vi "Aplicaderiva.vi"() -> ()   [LabVIEW 2010]
uses:
  <vilib>/Analysis/NI_AALPro.lvlib
panel:
  out "Waveform Chart 2":waveform(dbl)(graph)
  out "Waveform Chart":waveform(dbl)(graph)
  in  "stop":bool
  in  "Numeric":i32
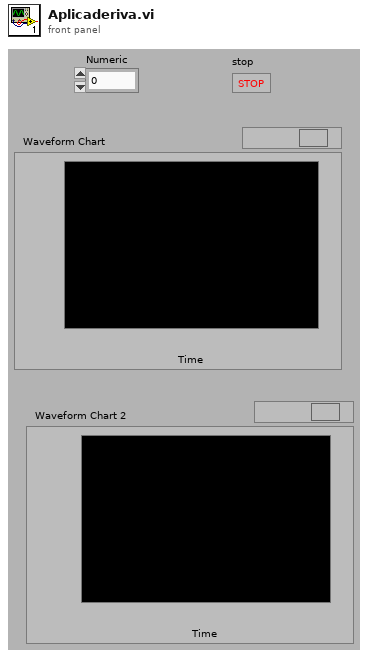
[diagram p1: front panel]
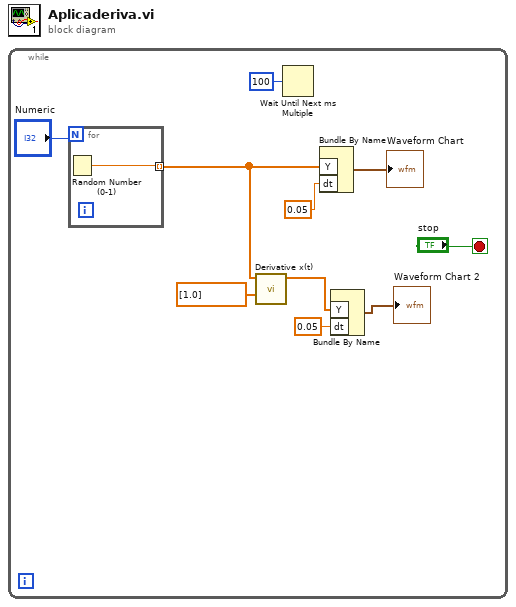
[diagram p0: block diagram]
diagram:
  n1 = while {
    stop <- "stop" stop-if-true
    n2 = for {
      N: "Numeric" -> [_]
      tunnel: [w11] -> w2 mode=indexing
      n3 = Random Number (0-1)() -> (number: 0 to 1=w11:dbl)
    }
    n4 = call <vilib>:"Derivative x(t).vi"("Final Condition"=dbl[] [1.0], "X"=w2) -> ("dX/dt"=w1:dbl[])  [unwired: 8 in, 1 out]
    n5 = Wait Until Next ms Multiple(millisecond multiple=u32 100) -> ()  [unwired: 1 out]
    n6 = Bundle By Name("Y"=w2, "dt"=0.05) -> (→"Waveform Chart":waveform(dbl))  [unwired: 1 in]
    n7 = Bundle By Name("Y"=w1, "dt"=0.05) -> (→"Waveform Chart 2":waveform(dbl))  [unwired: 1 in]
  }
